vi "Configure Generation.vi"(8 "error in":errorcluster, 11 "DO DAQmx Fixed Freq PWM CFG in":refnum<class "DO DAQmx Fixed Freq PWM CFG.lvclass">) -> (0 "error out":errorcluster, 3 "DO DAQmx Fixed Freq PWM CFG out":refnum<class "DO DAQmx Fixed Freq PWM CFG.lvclass">)   [LabVIEW 2024, in "DO DAQmx Fixed Freq PWM CFG.lvclass"]
uses:
  DO DAQmx Fixed Freq PWM CFG.lvclass
  D:/git/HAL/HAL/Configurations/CFG JSON/CFG JSON.lvclass
  D:/git/HAL/HAL/Configurations/CFG Base/CFG Base.lvclass
  D:/git/HAL/HAL/Devices/DAQmx/DAQmx Base CFG/DAQmx Base CFG.lvclass
  DAQmx Base CFG/DAQmx Base CFG.lvclass/DAQmx Base CFG.ctl
  Configurations/CFG Base/CFG Base.lvclass/CFG Base.ctl
  DO DAQmx Fixed Freq PWM CFG.lvclass/DO DAQmx Fixed Freq PWM CFG.ctl
  f180d75c-e615-46e4-b916-673f59557be0.vi
  <vilib>/DAQmx/write.llb/DAQmx Write (Digital 1D Wfm NChan NSamp).vi
  f180d75c-e615-46e4-b916-673f59557be0.vi/a4169a97-72fc-4003-a778-603cf20cafa0.vi
  <vilib>/JDP Science/JSONtext/Find Item.vi
  <vilib>/JDP Science/JSONtext/Next JSON Value.vi
  <vilib>/JDP Science/JSONtext/String Subset.vi
  <vilib>/JDP Science/JSONtext/Parsing/Advance past next JSON Value (inlined COPY).vi
  <vilib>/JDP Science/JSONtext/Parsing/Advance past whitespace.vi
  <vilib>/JDP Science/JSONtext/Parsing/Advance past String.vi
  <vilib>/JDP Science/JSONtext/Parsing/Advance past Number.vi
  <vilib>/JDP Science/JSONtext/Parsing/Advance past Line Ending.vi
  <vilib>/JDP Science/JSONtext/Parsing/Parse Full Path or Item Name.vi
  <vilib>/JDP Science/JSONtext/Parsing/Advance past Array.vi
  <vilib>/JDP Science/JSONtext/Parsing/Advance past Object.vi
  <vilib>/JDP Science/JSONtext/support/Error Cluster From Code.vi
  <vilib>/JDP Science/JSONtext/Offset/Find Item Locations by Path.vi
  <vilib>/JDP Science/JSONtext/JSON text to Variant.vi
  <vilib>/Utility/error.llb/Error Cluster From Error Code.vi
  <vilib>/Waveform/DWDTOps.llb/DWDT Uncompress Digital.vi
  <vilib>/DAQmx/miscellaneous.llb/DAQmx Fill In Error Info.vi
  <vilib>/JDP Science/JSONtext/LVClass Serializer/JSONtext LVClass Serializer.lvclass
  DAQmx Base CFG/DAQmx Base CFG.lvclass
  <resource>/objmgr/daqmx.rc
  Configurations/CFG JSON/CFG JSON.lvclass
  Configurations/CFG Base/CFG Base.lvclass
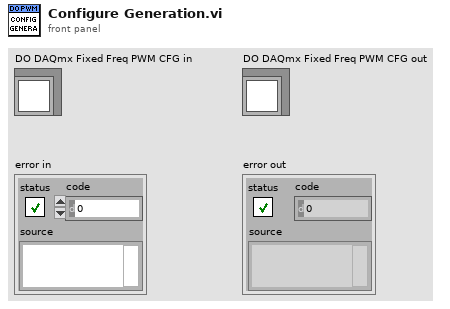
[diagram p1: front panel]
types:
  T1 = cluster{"Channel":string, "Digital Waveform":digitalwaveform}[]
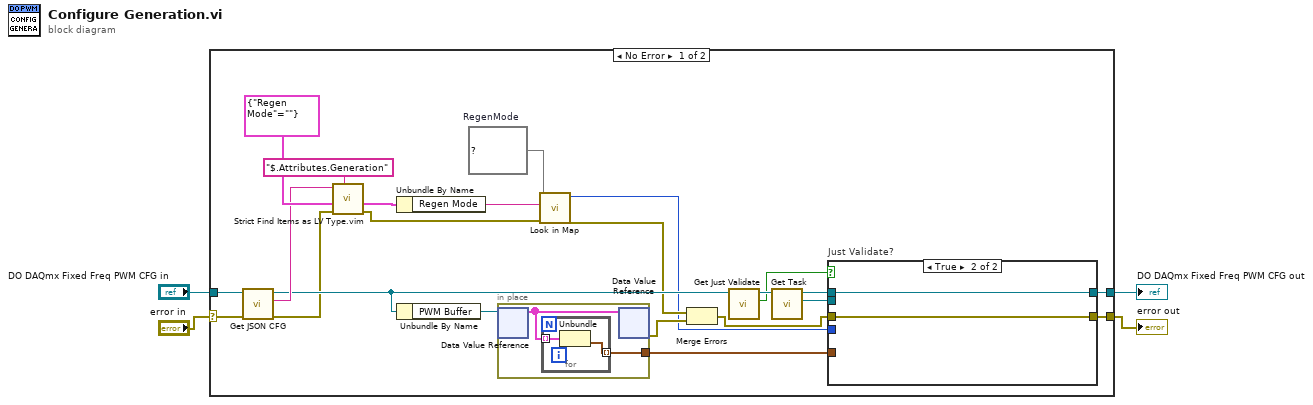
[diagram p0: block diagram]
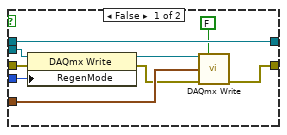
[diagram p2: hidden frame]
diagram:
  n1 = case shown="No Error" "error in" {
    selector: "error in" -> [w10 w43]
    tunnel: [w16 w43] -> w3
    tunnel: [w17 w42] -> w1
    tunnel: "DO DAQmx Fixed Freq PWM CFG in" -> [w25 w42]
    frame No Error {
      w9 = map{string, i32} {"Allow Regeneration"=10097, "Do Not Allow Regeneration"=10158}  # RegenMode
      n2 = call "Get JSON CFG.vi"("CFG JSON in"=w25) -> ("<JSON> CFG"=w21:string, "CFG JSON out"=w15:refnum<class "DO DAQmx Fixed Freq PWM CFG.lvclass">)  [unwired: 9 in]
      n3 = call "Strict Find Items as LV Type.vim"("$Path or Item Name"="$.Attributes.Generation", "error in"=w10, "Data Type and Default Value"=cluster{"Regen Mode":string} {"Regen Mode"=""}, "<JSON>"=w21) -> ("error out"=w5:errorcluster, "Data out"=w22:cluster{"Regen Mode":string})  [unwired: 5 in, 1 out]
      n4 = Unbundle By Name(w22) -> ("Regen Mode"=w8:string)
      n5 = Unbundle By Name(w15) -> ("PWM Buffer"=w14:refnum<data-value>)
      n6 = in-place {
        in-place-border: [w27] -> w13
        n7 = in-place-dvr #1(w14) -> (w28:T1)  [unwired: 1 out]
        n8 = for {
          tunnel: w28 -> [w30] mode=indexing
          tunnel: [w29] -> w27 mode=indexing
          n9 = Unbundle(w30) -> ("Digital Waveform"=w29:digitalwaveform)  [unwired: 1 out]
        }
        n10 = in-place-dvr #1(w28) -> (w12:errorcluster)  [unwired: 1 out]
      }
      n11 = call "Look in Map.vi"("error in"=w5, "Key"=w8, "Map"=w9) -> ("error out"=w7:errorcluster, "Value"=w6:i32)  [unwired: 7 in]
      n12 = Merge Errors(w7, w12) -> (w11:errorcluster)
      n13 = call "Get Just Validate.vi"("CFG Base in"=w15) -> ("Just Validate"=w19:bool, "CFG Base out"=w20:refnum<class "DO DAQmx Fixed Freq PWM CFG.lvclass">)  [unwired: 9 in]
      n14 = call "Get Task.vi"("DAQmx Base CFG in"=w20) -> ("Task"=w26:refnum<k21>, "DAQmx Base CFG out"=w18:refnum<class "DO DAQmx Fixed Freq PWM CFG.lvclass">)  [unwired: 9 in]
      n15 = case "Just Validate?" shown="True" w19 {
        tunnel: w11 -> [w39 w40]
        tunnel: w26 -> [w38 _]
        tunnel: w6 -> [w37 _]
        tunnel: w18 -> [w32 w41]
        tunnel: [w32 w41] -> w17
        tunnel: [w33 w40] -> w16
        tunnel: w13 -> [w35 _]
        frame False {
          n16 = property class="DAQmx Write"(reference=w38, error in=w39, "RegenMode"=w37) -> (reference out=w36:refnum<k21>, error out=w34:errorcluster)
          n17 = call-poly <vilib>:"DAQmx Write.vi"("task/channels in"=w36, "auto start"=FALSE, "data"=w35, "error in"=w34) -> ("error out"=w33:errorcluster)  [unwired: 9 in, 2 out]
        }
        frame True {
        }
      }
    }
    frame Error {
    }
  }
  "error out" <- w3
  "DO DAQmx Fixed Freq PWM CFG out" <- w1
